vi "Initialize Refs.vi"(0 "Current Device Address":u8, 1 "Name":string, 5 "Device Name":u64, 11 "error in (no error)":errorcluster) -> (4 "J1939 Cluster":T7, 6 "References":T1, 15 "error out":errorcluster)   [LabVIEW 2013, in "J1939 Addon Engine.lvlib"]
uses:
  Engine/J1939 Addon Engine.lvlib
  Types/Setup Information Cluster.ctl
  <vilib>/xnet/xnet.llb/XNET Frame CAN.ctl
  <vilib>/xnet/xnet.llb/XNET Frame Type CAN.ctl
  J1939 Utilities/Types/CAN Outgoing Message Cluster.ctl
  Types/TP List References.ctl
  Types/BAM Buffer Connections List_Ref.ctl
  Types/Connection Mode Generation Connection Ref.ctl
  Types/BAM Generation Connections List_Ref.ctl
  Types/Address Table Reference.ctl
  Types/RQST Lookup Table Reference.ctl
  J1939 Utilities/J1939 Utilities.lvlib
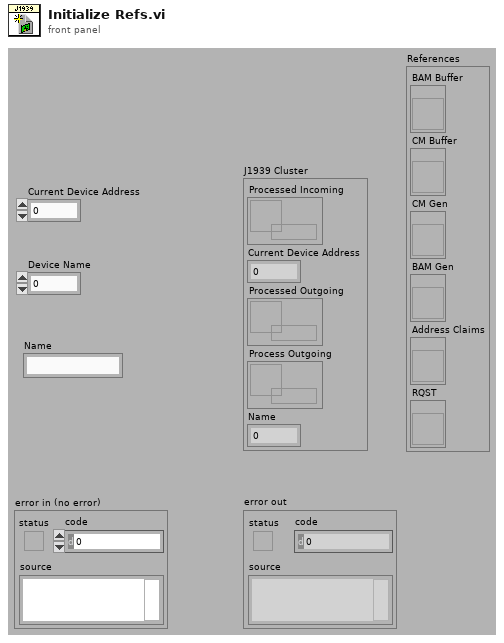
[diagram p1: front panel]
types:
  T1 = typedef "J1939 Addon Engine.lvlib/TP List References.ctl" = cluster{"BAM Buffer":T2, "CM Buffer":T2, "CM Gen":T3, "BAM Gen":T4, "Address Claims":T5, "RQST":T6}
  T2 = typedef "J1939 Addon Engine.lvlib/BAM Buffer Connections List_Ref.ctl" = refnum<vi>
  T3 = typedef "J1939 Addon Engine.lvlib/Connection Mode Generation Connection Ref.ctl" = refnum<vi>
  T4 = typedef "J1939 Addon Engine.lvlib/BAM Generation Connections List_Ref.ctl" = refnum<vi>
  T5 = typedef "J1939 Addon Engine.lvlib/Address Table Reference.ctl" = refnum<vi>
  T6 = typedef "J1939 Addon Engine.lvlib/RQST Lookup Table Reference.ctl" = refnum<vi>
  T7 = typedef "J1939 Addon Engine.lvlib/Setup Information Cluster.ctl" = cluster{"Processed Incoming":refnum<queue>, "Current Device Address":u8, "Processed Outgoing":refnum<queue>, "Process Outgoing":refnum<queue>, "Name":u64}
  T8 = typedef "XNET Frame CAN.ctl" = cluster{"timestamp":timestamp, "payload":u8[], "identifier":u32, "type":T9, "extended?":bool, "echo?":bool}
  T9 = typedef "XNET Frame Type CAN.ctl" = u8
  T10 = typedef "J1939 Utilities.lvlib/CAN Outgoing Message Cluster.ctl" = cluster{"Identifier":u32, "Data":u8[]}
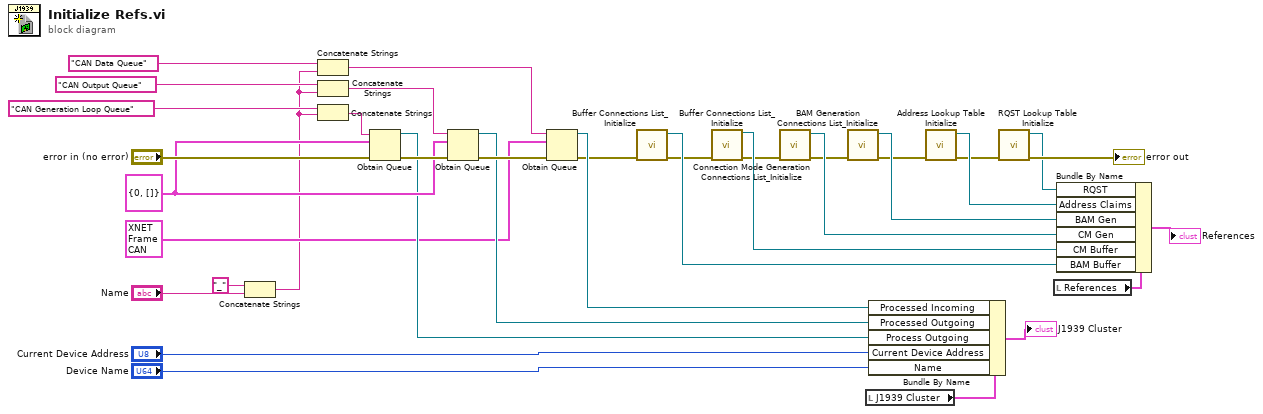
[diagram p0: block diagram]
diagram:
  w29 = T10 {"Identifier"=0, "Data"=[]} ("Data to Send")
  n1 = Concatenate Strings("_", "Name") -> (w2:string)
  n2 = Concatenate Strings("CAN Data Queue" ("name (unnamed)"), w2) -> (w7:string)
  n3 = Concatenate Strings("CAN Output Queue" ("name (unnamed)"), w2) -> (w5:string)
  n4 = Concatenate Strings("CAN Generation Loop Queue" ("name (unnamed)"), w2) -> (w3:string)
  n5 = Obtain Queue(name (unnamed)=w3, element data type=w29, error in (no error)="error in (no error)") -> (queue out=w28:refnum<queue>, error out=w34:errorcluster)  [unwired: 2 in, 1 out]
  n6 = Obtain Queue(name (unnamed)=w5, element data type=w29, error in (no error)=w34) -> (queue out=w30:refnum<queue>, error out=w33:errorcluster)  [unwired: 2 in, 1 out]
  n7 = Obtain Queue(name (unnamed)=w7, element data type=T8 {"timestamp"=timestamp(0 s since 1904-01-01), "payload"=[], "identifier"=0, "type"=0, "extended?"=FALSE, "echo?"=FALSE} ("CAN frame"), error in (no error)=w33) -> (queue out=w31:refnum<queue>, error out=w26:errorcluster)  [unwired: 2 in, 1 out]
  n8 = call "Buffer Connections List_Initialize.vi"("error in (no error)"=w26) -> ("error out"=w22:errorcluster, "reference out"=w24:T2)  [unwired: 9 in]
  n9 = call "Buffer Connections List_Initialize.vi"("error in (no error)"=w22) -> ("error out"=w20:errorcluster, "reference out"=w21:T2)  [unwired: 9 in]
  n10 = call "Connection Mode Generation Connections List_Initialize.vi"("error in (no error)"=w20) -> ("error out"=w18:errorcluster, "CM Gen Ref out"=w19:T3)  [unwired: 9 in]
  n11 = call "BAM Generation Connections List_Initialize.vi"("error in (no error)"=w18) -> ("error out"=w16:errorcluster, "BAM Gen"=w17:T4)  [unwired: 9 in]
  n12 = local read "J1939 Cluster"() -> (w32:T7)
  n13 = Bundle By Name(cluster=w32, "Processed Incoming"=w31, "Processed Outgoing"=w30, "Process Outgoing"=w28, "Current Device Address"="Current Device Address", "Name"="Device Name") -> (→"J1939 Cluster":T7)
  n14 = call "Address Lookup Table Initialize.vi"("error in (no error)"=w16) -> ("error out"=w13:errorcluster, "reference out 2"=w15:T5)  [unwired: 9 in]
  n15 = call "RQST Lookup Table Initialize.vi"("error in (no error)"=w13) -> ("error out"=→"error out":errorcluster, "reference out"=w11:T6)  [unwired: 9 in]
  n16 = local read "References"() -> (w25:T1)
  n17 = Bundle By Name(cluster=w25, "RQST"=w11, "Address Claims"=w15, "BAM Gen"=w17, "CM Gen"=w19, "CM Buffer"=w21, "BAM Buffer"=w24) -> (→"References":T1)
